vi "Find All Log Files.vi"(8 "error in":errorcluster, 11 "embedded data logger in":T1=18446744073709551615 format="%.0x") -> (0 "error out":errorcluster, 2 "log files":T1[](array[typedef]) format="%.0x", 3 "embedded data logger out":T1 format="%.0x")   [LabVIEW 2027, in "Embedded Data Logger Scripting.lvlib"]
uses:
  Embedded Data Logger Scripting.lvlib
  <vilib>/NI VeriStand/Custom Device API/Custom Device Item Ref.ctl
  Shared/Constants.vi
  <vilib>/NI VeriStand/Custom Device Tools/Custom Device Utility Library/NI VeriStand - Search for All Items by GUID.vi
  <vilib>/NI VeriStand/Custom Device Tools/Custom Device Utility Library/Custom Device Utility Library.lvlib
  Shared/Embedded Data Logger Shared.lvlib
  <vilib>/NI VeriStand/Custom Device API/Custom Device API.lvlib
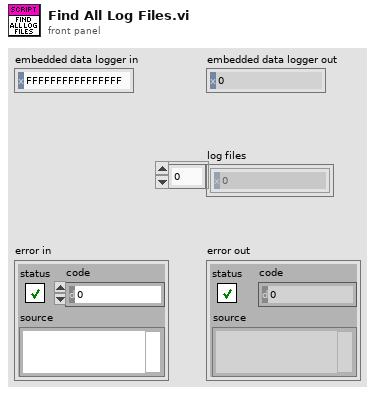
[diagram p1: front panel]
types:
  T1 = typedef "Custom Device API.lvlib/Custom Device Item Ref.ctl" = u64
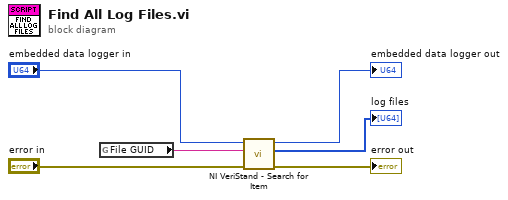
[diagram p0: block diagram]
diagram:
  n1 = global read "Constants.vi" "File GUID"() -> (w2:string)
  n2 = call-poly <vilib>:"NI VeriStand - Search for Item.vi"("error in"="error in", "Item GUID"=w2, "Section Ref in"="embedded data logger in") -> ("error out"=→"error out":errorcluster, "Item Refs"=→"log files":T1[], "Section Ref out"=→"embedded data logger out":T1)  [unwired: 5 in, 1 out]
